vi "LaunchEditor.vi"(8 "error in (no error)":errorcluster {"code" format="Error %.0f"}, 10 "Editor Events":T1, 11 "VIDocEditor in":refnum<class "VIDocEditor.lvclass">) -> (0 "error out":errorcluster {"code" format="Error %.0f"}, 2 "VI Refnum":refnum<vi>, 3 "VIDocEditor out":refnum<class "VIDocEditor.lvclass">)   [LabVIEW 2023, in "VIDocEditor.lvclass"]
uses:
  VIDocEditor.lvclass
  Editor Events Cluster.ctl
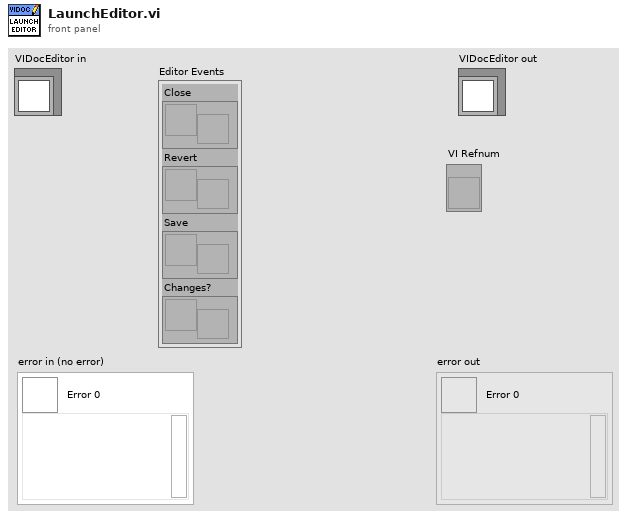
[diagram p1: front panel]
types:
  T1 = typedef "VIDocEditor.lvclass/Editor Events Cluster.ctl" = cluster{"Close":refnum<user-event>, "Revert":refnum<user-event>, "Save":refnum<user-event>, "Changes?":refnum<user-event>}
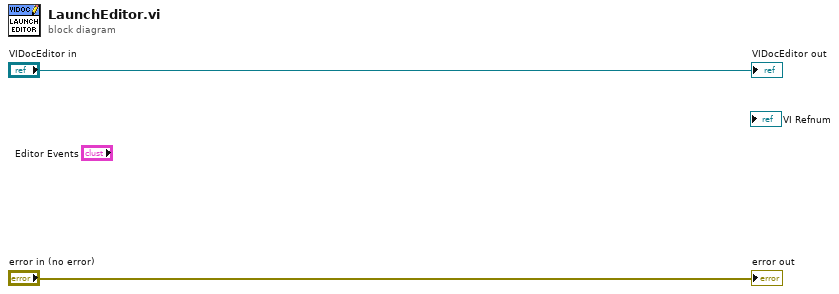
[diagram p0: block diagram]
diagram:
  "error out" <- "error in (no error)"
  "VIDocEditor out" <- "VIDocEditor in"
